vi "DelayProject_WedgeDelay.vi"() -> ()   [LabVIEW 2019]
uses:
  Delete/Control 7.ctl
  Delete/Control 2.ctl
  Delete/Control 1.ctl
  Delete/Control 3.ctl
  Delete/Control 6.ctl
  Delete/Control 4.ctl
  Delete/Control 5.ctl
  Delete/Control 8.ctl
  C:/DATA/Megan/LabviewScripts/ThorlabsKinesisDrivers/Thorlabs.MotionControl.TCube.DCServoCLI.dll
  Thorlabs.MotionControl.TCube.DCServoCLI.dll
  C:/DATA/Megan/LabviewScripts/ThorlabsKinesisDrivers/Thorlabs.MotionControl.Controls.dll
  Thorlabs.MotionControl.Controls.dll
  Program Files (x86)/National Instruments/LabVIEW 2011/user.lib/Nanonis Prog Interface/Nanonis Prog Interface.lvlib
panel:
  in  "TCubeDCServoControl":refnum<k24>(container)
  in  "Start Move B":bool
  in  "Set Position B (mm)":T1 format="%.3f"
  in  "Clear Plots":bool
  in  "Data3":dbl[][](array[numeric])
  out "AFM":cluster{dbl[], dbl[]}[](graph)
  in  "Data2":dbl[][](array[numeric])
  in  "Data1":dbl[][](array[numeric])
  in  "Plot3":bool
  in  "Plot2":bool
  in  "Plot1":bool
  out "Optics":cluster{dbl[], dbl[]}[](graph)
  out "Array":string[][](array[string])
  in  "AC bias (Hz)":string
  in  "AC bias":string
  in  "DC bias":string
  in  "Tip lift":string
  in  "Time const":string
  in  "Prop gain":string
  in  "Polarization":string
  in  "Notes":string
  in  "Location":string
  out "AC bias (Hz)":string="AC Bias (Hz)"
  out "AC bias":string="AC Bias (V)"
  out "DC bias":string="DC Bias (V)"
  out "Polarization":string="Polarization (deg)"
  out "Tip Lift":string="Tip Lift"
  out "Notes":string="Notes"
  out "Location":string="Location"
  out "Time Const":string="Time constant (s)"
  out "Prop Gain":string="Proportional gain (m/Hz)"
  in  "Net Power":string
  in  "Wavelength":string
  out "Net Power":string="Net power (mW)"
  out "Wavelength":string="Wavelength (nm)"
  out "Instantaneous":dbl
  in  "Channel":dbl
  out "Average":dbl
  in  "Wait After (ms)":T2=100.0
  in  "Wait Before (ms)":T3=100.0
  in  "Points per Step":T4=10.0
  in  "Save Sweep":bool
  out "Total Time (min:sec)":string
  out "Range (fs)":dbl
  out "Total Distance (mm)":dbl
  in  "Step Size (mm)":T5 format="%.4f"
  in  "Start Position (mm)":T6=80.0
  in  "End Position (mm)":T7=90.0
  out "Step Size (fs)":dbl=100.0
  out "Status":string
  in  "Set Position A (mm)":T8 format="%.3f"
  in  "Start Move A":bool
  in  "Start Sweep":bool
  out "Time Remaining (min:sec)":string
  in  "Stop Sweep":bool
  out "Position  (mm)":ext format="%.3f"
  # "Wedge Delay"
  # "Sweep"
  # "This program moves the MTS50-Z8 translational delay stage either in a single step (Move), or a  stepped sweep (Sweep). \n\nThe sequence of events in the Sweep is as follows:\n1) Home the stage.\n2) Go to the Start Position; wait 1s.\n3) Move by Step Size.\n4)  Wait Before time. \n5) Write Position to Nanonis Output 8.\n6) Read all Nanonis Channels, Points per Step times.\n7) Take the average of these instantaneous readouts.\n8) Wait After time.\n9) Repeat 3-8 for each step. \n10) Save all Nanonis channels and record Attributes in header.\n\nThe Readouts are for this VI display only, to visualize what the program is doing. Channel is the Nanonis channel displayed. \n\nIf the Set/Start/End positions are outside of the operating range [-1:50]mm, the Move/Sweep will not execute. Short wait times may lead to errors if  they don't allow time  to move. \n\nThis VI needs to be opened from the project directory. This project and VI need to be in the same directory as the Thorlabs Kinesis folder, and require a 64-bit version of Labview. This program cannot run simultaneously with AirDelay.vi"
  # "Attributes"
  # "Parameters"
  # "Readouts"
  # "Move A"
  # "Move B"
  # "Air Delay: 93.15 mm"
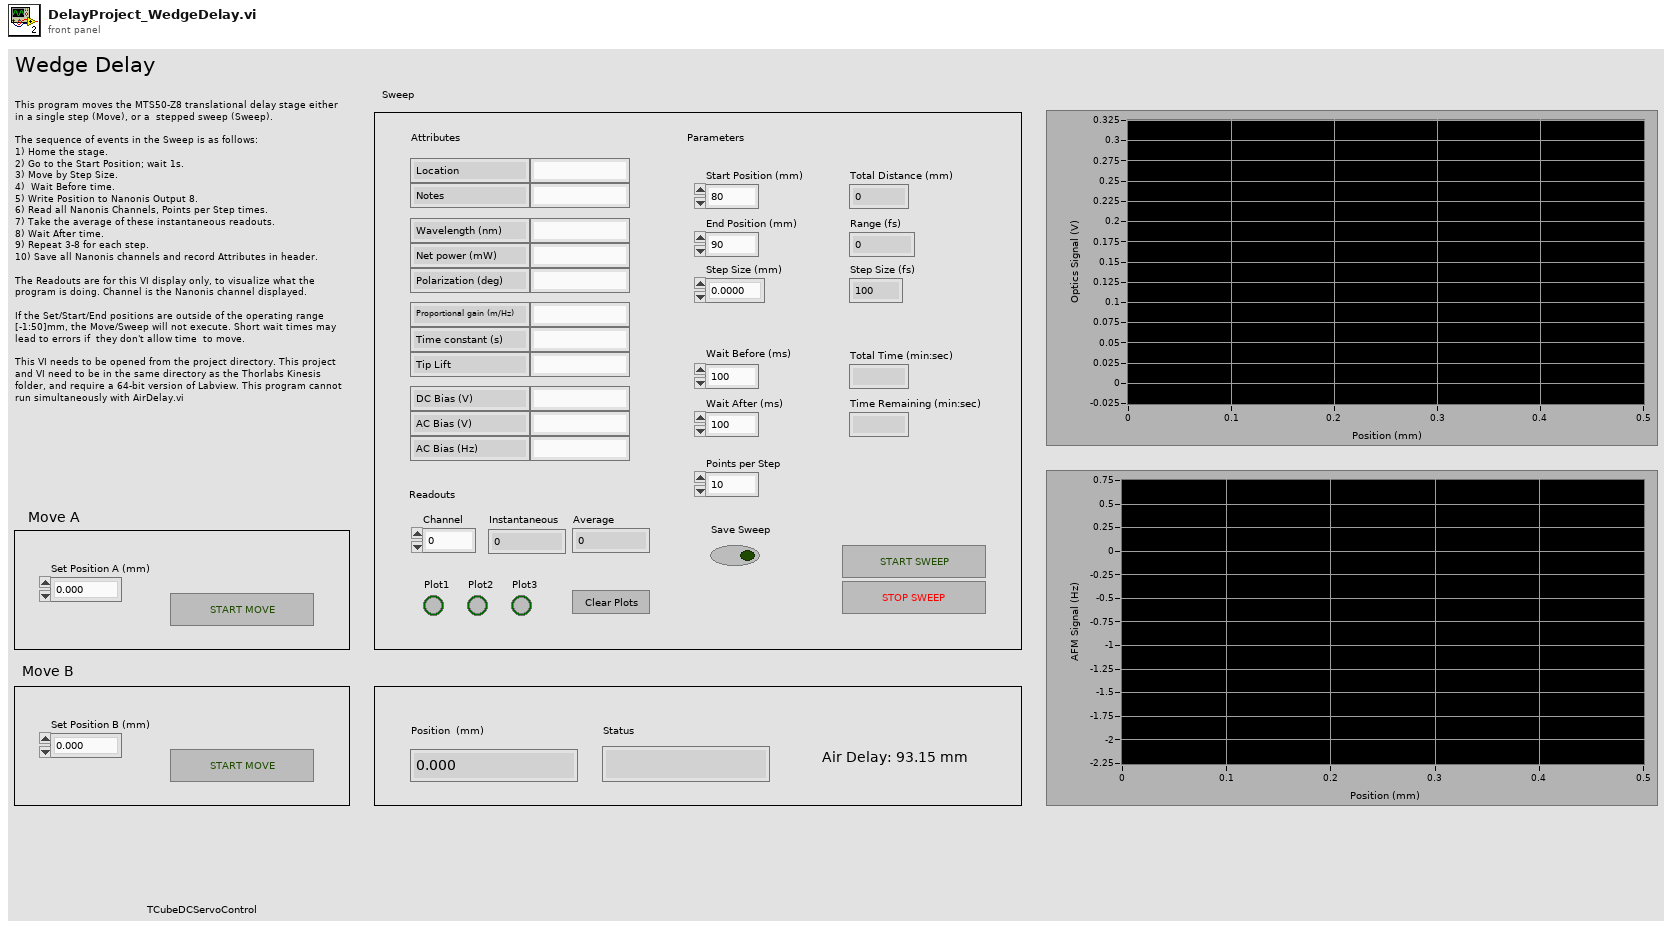
[diagram p1: front panel]
types:
  T1 = typedef "Control 8.ctl" = ext
  T2 = typedef "Control 5.ctl" = dbl
  T3 = typedef "Control 4.ctl" = dbl
  T4 = typedef "Control 6.ctl" = dbl
  T5 = typedef "Control 3.ctl" = dbl
  T6 = typedef "Control 1.ctl" = dbl
  T7 = typedef "Control 2.ctl" = dbl
  T8 = typedef "Control 7.ctl" = ext
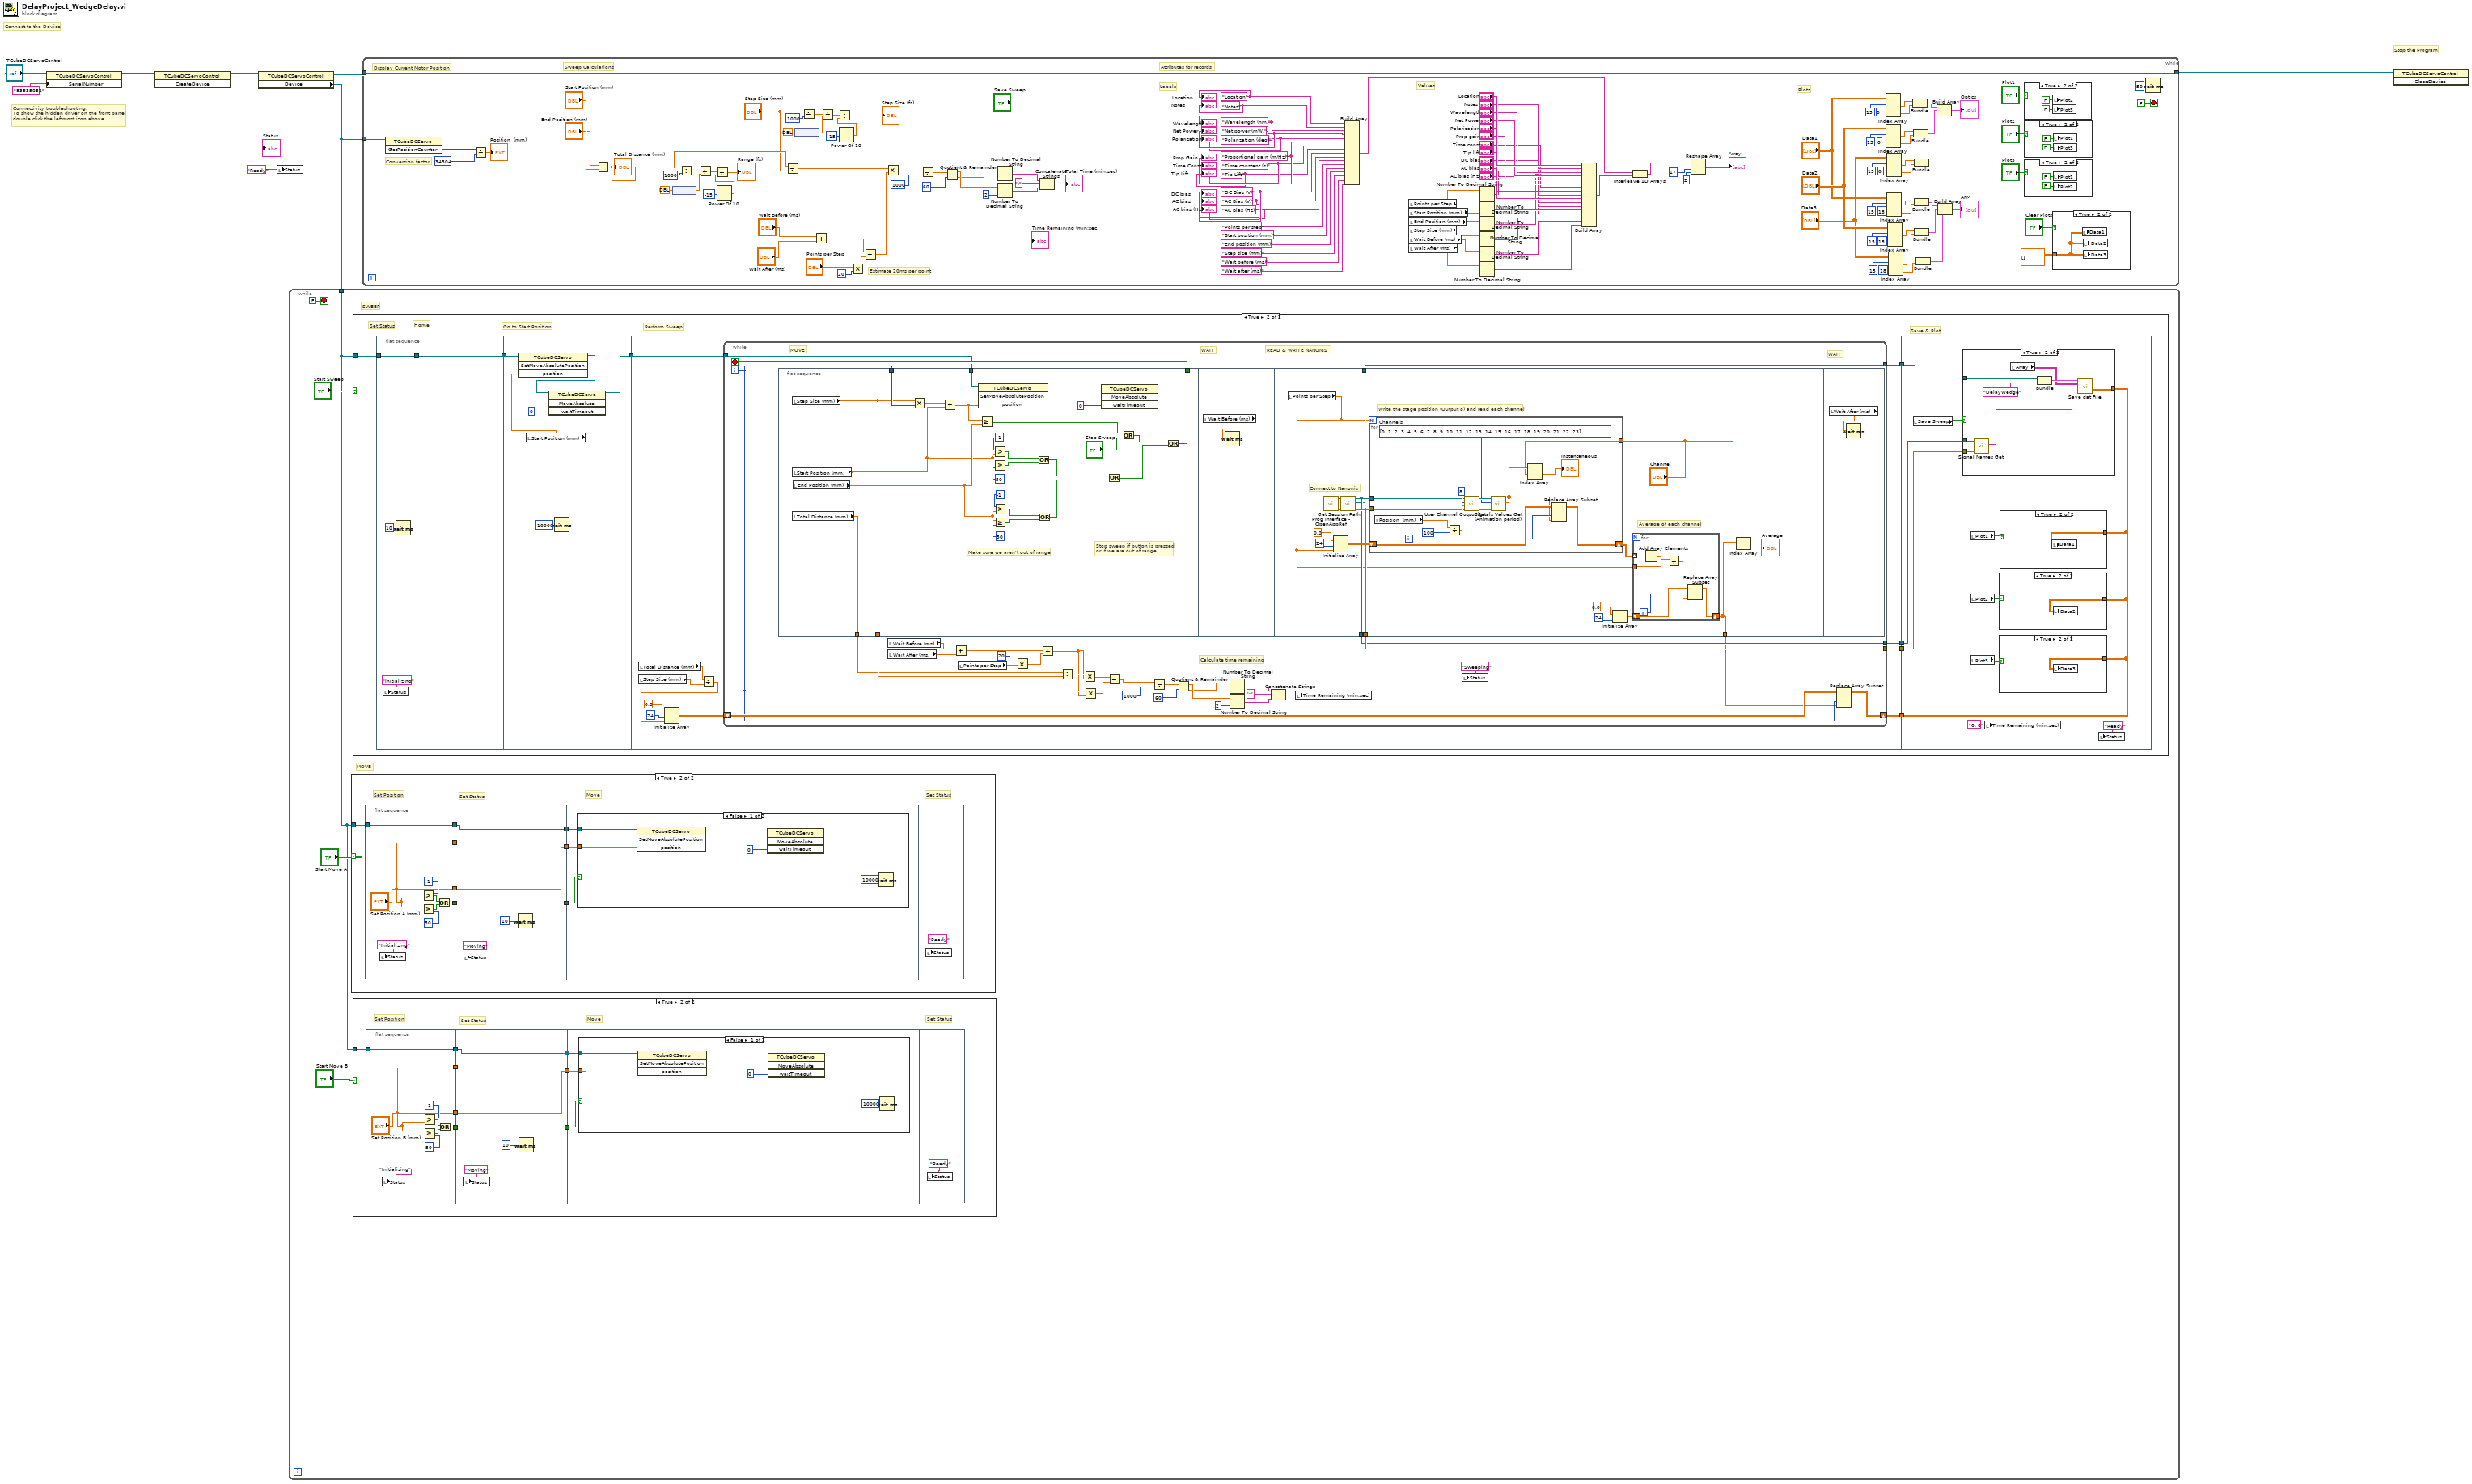
[diagram p0: block diagram]
diagram:
  # "Connectivity troubleshooting: \nTo show the hidden driver on the front panel \ndouble click the leftmost icon above."
  # "Stop the Program"
  # "Connect to the Device"
  n1 = property class="TCubeDCServoControl"(reference="TCubeDCServoControl", "SerialNumber"="83835052") -> (reference out=w8:refnum<k24>)  [unwired: 1 in, 1 out]
  n2 = invoke class="TCubeDCServoControl" method="CreateDevice"(reference=w8) -> (reference out=w5:refnum<k24>)  [unwired: 2 in, 2 out]
  n3 = property class="TCubeDCServoControl"(reference=w5) -> (reference out=w4:refnum<k24>, "Device"=w3:refnum<k24>)  [unwired: 1 in, 1 out]
  n4 = local write "Status"("Ready") -> ()
  n5 = while {
    tunnel: w3 -> [w9]
    stop <- FALSE stop-if-true
    # "MOVE"
    # "SWEEP"
    n6 = case shown="True" "Start Move A" {
      tunnel: w9 -> [_ w51]
      frame False {
      }
      frame True {
        # "Set Status"
        # "Move"
        # "Set Status"
        # "Set Position"
        n7 = flat-sequence {
          tunnel: w51 -> [w59]
          tunnel: [w59] -> w50
          tunnel: ["Set Position A (mm)"] -> w49
          tunnel: [w53] -> w48
          tunnel: ["Set Position A (mm)"] -> w45
          tunnel: w50 -> [w62]
          tunnel: w49 -> [_]
          tunnel: w48 -> [w64]
          tunnel: [w64] -> w47
          tunnel: [w63] -> w46
          tunnel: w45 -> [w63]
          tunnel: [w62] -> w44
          tunnel: w47 -> [w67]
          tunnel: w46 -> [w66]
          tunnel: w44 -> [w65]
          frame #0 {
            n8 = local write "Status"("Initializing") -> ()
            n9 = Greater?(x=-1, y="Set Position A (mm)") -> (0:w58:bool)
            n10 = Greater Or Equal?(x="Set Position A (mm)", y=50) -> (x >= y?=w57:bool)
            n11 = Or(x=w58, y=w57) -> (x .or. y?=w53:bool)
          }
          frame #1 {
            n12 = local write "Status"("Moving") -> ()
            n13 = Wait (ms)(milliseconds to wait=10) -> ()  [unwired: 1 out]
          }
          frame #2 {
            n14 = case shown="False" w67 {
              tunnel: w66 -> [w69 _]
              tunnel: w65 -> [w70 _]
              frame False {
                n15 = invoke class="TCubeDCServo" method="SetMoveAbsolutePosition"(reference=w70, "position"=w69) -> (reference out=w72:refnum<k24>)  [unwired: 2 in, 3 out]
                n16 = invoke class="TCubeDCServo" method="MoveAbsolute"(reference=w72, "waitTimeout"=0) -> ()  [unwired: 2 in, 4 out]
                n17 = Wait (ms)(milliseconds to wait=10000) -> ()  [unwired: 1 out]
              }
              frame True {
              }
            }
          }
          frame #3 {
            n18 = local write "Status"("Ready") -> ()
          }
        }
      }
    }
    n19 = case shown="True" "Start Move B" {
      tunnel: w9 -> [_ w21]
      frame False {
      }
      frame True {
        # "Set Status"
        # "Move"
        # "Set Status"
        # "Set Position"
        n20 = flat-sequence {
          tunnel: w21 -> [w29]
          tunnel: [w29] -> w20
          tunnel: ["Set Position B (mm)"] -> w19
          tunnel: [w24] -> w18
          tunnel: ["Set Position B (mm)"] -> w15
          tunnel: w20 -> [w32]
          tunnel: w19 -> [_]
          tunnel: w18 -> [w34]
          tunnel: [w34] -> w17
          tunnel: [w33] -> w16
          tunnel: w15 -> [w33]
          tunnel: [w32] -> w14
          tunnel: w17 -> [w37]
          tunnel: w16 -> [w36]
          tunnel: w14 -> [w35]
          frame #0 {
            n21 = local write "Status"("Initializing") -> ()
            n22 = Greater?(x=-1, y="Set Position B (mm)") -> (0:w28:bool)
            n23 = Greater Or Equal?(x="Set Position B (mm)", y=50) -> (x >= y?=w27:bool)
            n24 = Or(x=w28, y=w27) -> (x .or. y?=w24:bool)
          }
          frame #1 {
            n25 = local write "Status"("Moving") -> ()
            n26 = Wait (ms)(milliseconds to wait=10) -> ()  [unwired: 1 out]
          }
          frame #2 {
            n27 = case shown="False" w37 {
              tunnel: w36 -> [w39 _]
              tunnel: w35 -> [w40 _]
              frame False {
                n28 = invoke class="TCubeDCServo" method="SetMoveAbsolutePosition"(reference=w40, "position"=w39) -> (reference out=w42:refnum<k24>)  [unwired: 2 in, 3 out]
                n29 = invoke class="TCubeDCServo" method="MoveAbsolute"(reference=w42, "waitTimeout"=0) -> ()  [unwired: 2 in, 4 out]
                n30 = Wait (ms)(milliseconds to wait=10000) -> ()  [unwired: 1 out]
              }
              frame True {
              }
            }
          }
          frame #3 {
            n31 = local write "Status"("Ready") -> ()
          }
        }
      }
    }
    n32 = case shown="True" "Start Sweep" {
      tunnel: w9 -> [_ w81]
      frame False {
      }
      frame True {
        # "Save & Plot"
        # "Set Status"
        # "Perform Sweep"
        # "Go to Start Position"
        # "Home"
        n33 = flat-sequence {
          tunnel: w81 -> [w84]
          tunnel: [w84] -> w80
          tunnel: [w85] -> w79
          tunnel: w80 -> [w85]
          tunnel: w79 -> [w91]
          tunnel: [w88] -> w78
          tunnel: w78 -> [w102]
          tunnel: [w101] -> w77
          tunnel: [w100] -> w76
          tunnel: [w99] -> w75
          tunnel: [w92] -> w74
          tunnel: w77 -> [w208]
          tunnel: w76 -> [w207]
          tunnel: w75 -> [w206]
          tunnel: w74 -> [w204]
          frame #0 {
            n34 = local write "Status"("Initializing") -> ()
            n35 = Wait (ms)(milliseconds to wait=10) -> ()  [unwired: 1 out]
          }
          frame #1 {
          }
          frame #2 {
            n36 = local read "Start Position (mm)"() -> (w86:T6)
            n37 = invoke class="TCubeDCServo" method="SetMoveAbsolutePosition"(reference=w91, "position"=w86) -> (reference out=w89:refnum<k24>)  [unwired: 2 in, 3 out]
            n38 = invoke class="TCubeDCServo" method="MoveAbsolute"(reference=w89, "waitTimeout"=0) -> (reference out=w88:refnum<k24>)  [unwired: 2 in, 3 out]
            n39 = Wait (ms)(milliseconds to wait=10000) -> ()  [unwired: 1 out]
          }
          frame #3 {
            n40 = local read "Total Distance (mm)"() -> (w96:dbl)
            n41 = local read "Step Size (mm)"() -> (w95:T5)
            n42 = Divide(x=w96, y=w95) -> (x/y=w94:T5)
            n43 = Initialize Array(0.0, 24, w94) -> (w93:dbl[][])
            n44 = while {
              tunnel: w102 -> [w134]
              tunnel: [w114] -> w101
              tunnel: [w115] -> w100
              tunnel: [w113] -> w99
              shift-right: [w109] -> w92
              shift-left: w93 -> [w112]
              i -> [w111]
              stop <- w135 stop-if-true
              # "WAIT"
              # "READ & WRITE NANONIS"
              # "WAIT"
              # "MOVE"
              # "Calculate time remaining"
              n45 = flat-sequence {
                tunnel: w111 -> [w140]
                tunnel: [w139] -> w135
                tunnel: w134 -> [w138]
                tunnel: [w137] -> w124
                tunnel: [w136] -> w123
                tunnel: [w167] -> w115
                tunnel: [w166] -> w114
                tunnel: [w165] -> w113
                tunnel: [w164] -> w110
                frame #0 {
                  # "Stop sweep if button is pressed\nor if we are out of range"
                  # "Make sure we aren't out of range"
                  n46 = local read "Step Size (mm)"() -> (w137:T5)
                  n47 = local read "Start Position (mm)"() -> (w159:T6)
                  n48 = local read "Total Distance (mm)"() -> (w136:dbl)
                  n49 = local read "End Position (mm)"() -> (w160:T7)
                  n50 = Multiply(x=w137, y=w140) -> (x*y=w145:T5)
                  n51 = Add(x=w145, y=w159) -> (x+y=w146:T5)
                  n52 = invoke class="TCubeDCServo" method="SetMoveAbsolutePosition"(reference=w138, "position"=w146) -> (reference out=w141:refnum<k24>)  [unwired: 2 in, 3 out]
                  n53 = Greater Or Equal?(x=w146, y=w160) -> (x >= y?=w144:bool)
                  n54 = Greater?(x=-1, y=w159) -> (0:w151:bool)
                  n55 = Greater Or Equal?(x=w159, y=50) -> (x >= y?=w152:bool)
                  n56 = Greater?(x=-1, y=w160) -> (0:w155:bool)
                  n57 = Greater Or Equal?(x=w160, y=50) -> (x >= y?=w156:bool)
                  n58 = Or(x=w151, y=w152) -> (x .or. y?=w157:bool)
                  n59 = Or(x=w155, y=w156) -> (x .or. y?=w158:bool)
                  n60 = invoke class="TCubeDCServo" method="MoveAbsolute"(reference=w141, "waitTimeout"=0) -> ()  [unwired: 2 in, 4 out]
                  n61 = Or(x=w157, y=w158) -> (x .or. y?=w148:bool)
                  n62 = Or(x=w144, y="Stop Sweep") -> (x .or. y?=w147:bool)
                  n63 = Or(x=w147, y=w148) -> (x .or. y?=w139:bool)
                }
                frame #1 {
                  n64 = local read "Wait Before (ms)"() -> (w161:T3)
                  n65 = Wait (ms)(milliseconds to wait=w161) -> ()  [unwired: 1 out]
                }
                frame #2 {
                  # "Write the stage position (Output 8) and read each channel"
                  # "Average of each channel"
                  # "Connect to Nanonis"
                  n66 = local read "Points per Step"() -> (w163:T4)
                  n67 = call "Prog Interface - OpenAppRef.vi"() -> ("Error out"=w168:errorcluster, "Application reference"=w169:refnum<vi>)  [unwired: 6 in]
                  n68 = Initialize Array(0.0, 24, w163) -> (w172:dbl[][])
                  n69 = call "Get Session Path.vi"("error in (no error)"=w168, "Application ref in"=w169) -> ("error out"=w167:errorcluster, "Session path"=w165:path, "Application ref out"=w166:refnum<vi>)  [unwired: 7 in]
                  n70 = for {
                    N: w163 -> [_]
                    tunnel: w167 -> [w193]
                    tunnel: w166 -> [w192]
                    shift-right: [w191] -> w176
                    shift-left: w172 -> [w190]
                    tunnel: "Channel" -> [w185]
                    i -> [w189]
                    w186 = i32[] [0, 1, 2, 3, 4, 5, 6, 7, 8, 9, 10, 11, 12, 13, 14, 15, 16, 17, 18, 19, 20, 21, 22, 23]  # Channels
                    n71 = local read "Position  (mm)"() -> (w187:ext)
                    n72 = Divide(x=w187, y=100) -> (x/y=w196:ext)
                    n73 = call "User Channel Output Set.vi"("error in (no error)"=w193, "Output value (physical unit)"=w196, "User output channel (1-8)"=8, "Application ref in"=w192) -> ("error out"=w198:errorcluster, "Application ref out"=w197:refnum<vi>)  [unwired: 5 in]
                    n74 = call "Signals Values Get (Animation period).vi"("error in (no error)"=w198, "Signals indexes (0-23)"=w186, "Application ref in"=w197) -> ("Signals Values"=w188:sgl[])  [unwired: 5 in, 2 out]
                    n75 = Index Array(array=w188, index #1=w185) -> (element #1=→"Instantaneous":sgl)  [unwired: 1 in, 1 out]
                    n76 = Replace Array Subset(array=w190, new element=w188, index (col)=w189) -> (w191:dbl[][])  [unwired: 1 in]
                  }
                  n77 = Initialize Array(0.0, 24) -> (w175:dbl[])
                  n78 = for {
                    tunnel: w163 -> [w184]
                    tunnel: w176 -> [w180] mode=indexing
                    shift-right: [w182] -> w164
                    shift-left: w175 -> [w183]
                    i -> [w181]
                    n79 = Add Array Elements(numeric array=w180) -> (sum=w178:dbl)
                    n80 = Divide(x=w178, y=w184) -> (x/y=w179:T4)
                    n81 = Replace Array Subset(array=w183, new element=w179, index=w181) -> (w182:dbl[])
                  }
                  n82 = Index Array(array=w164, index="Channel") -> (element=→"Average":dbl)
                }
                frame #3 {
                  n83 = local read "Wait After (ms)"() -> (w200:T2)
                  n84 = Wait (ms)(milliseconds to wait=w200) -> ()  [unwired: 1 out]
                }
              }
              n85 = local read "Wait Before (ms)"() -> (w117:T3)
              n86 = local read "Wait After (ms)"() -> (w116:T2)
              n87 = Add(x=w117, y=w116) -> (x+y=w107:T3)
              n88 = local read "Points per Step"() -> (w108:T4)
              n89 = Multiply(x=20, y=w108) -> (x*y=w105:T4)
              n90 = Add(x=w107, y=w105) -> (x+y=w106:T3)
              n91 = Divide(x=w123, y=w124) -> (x/y=w125:T5)
              n92 = Multiply(x=w125, y=w106) -> (x*y=w126:T5)
              n93 = Multiply(x=w111, y=w106) -> (x*y=w128:T3)
              n94 = Subtract(x=w126, y=w128) -> (x-y=w127:T5)
              n95 = Divide(x=w127, y=1000) -> (x/y=w133:T5)
              n96 = Quotient & Remainder(x=w133, y=60) -> (x-y*floor(x/y)=w132:T5, floor(x/y)=w131:T5)
              n97 = Number To Decimal String(number=w131) -> (decimal integer string=w130:string)  [unwired: 1 in]
              n98 = Number To Decimal String(number=w132, width (-)=2) -> (decimal integer string=w129:string)
              n99 = Concatenate Strings(w130, ":", w129) -> (w103:string)
              n100 = local write "Time Remaining (min:sec)"(w103) -> ()
              n101 = local write "Status"("Sweeping") -> ()
              n102 = Replace Array Subset(array=w112, new element=w110, index (col)=w111) -> (w109:dbl[][])  [unwired: 1 in]
            }
          }
          frame #4 {
            n103 = local read "Save Sweep"() -> (w209:bool)
            n104 = case shown="True" w209 {
              tunnel: w207 -> [_ w219]
              tunnel: w208 -> [_ w218]
              tunnel: w206 -> [_ w216]
              tunnel: w204 -> [_ w215]
              frame False {
              }
              frame True {
                n105 = call "Signal Names Get.vi"("error in (no error)"=w219, "Application ref in"=w218) -> ("Signals Names"=w217:string[])  [unwired: 5 in, 2 out]
                n106 = local read "Array"() -> (w214:string[][])
                n107 = Bundle("Session path"=w216, "DelayWedge") -> (w221:cluster{"Session path":path, string})  [unwired: 1 in]
                n108 = call "Save dat File.vi"("Filename control"=w221, "Attributes"=w214, "Channels names"=w217, "Data"=w215) -> ()  [unwired: 8 in, 4 out]
              }
            }
            n109 = local read "Plot1"() -> (w201:bool)
            n110 = local read "Plot2"() -> (w202:bool)
            n111 = local read "Plot3"() -> (w203:bool)
            n112 = local write "Time Remaining (min:sec)"("0: 0") -> ()
            n113 = case shown="True" w202 {
              tunnel: w204 -> [_ w212]
              frame False {
              }
              frame True {
                n114 = local write "Data2"(w212) -> ()
              }
            }
            n115 = case shown="True" w203 {
              tunnel: w204 -> [_ w211]
              frame False {
              }
              frame True {
                n116 = local write "Data3"(w211) -> ()
              }
            }
            n117 = case shown="True" w201 {
              tunnel: w204 -> [_ w213]
              frame False {
              }
              frame True {
                n118 = local write "Data1"(w213) -> ()
              }
            }
            n119 = local write "Status"("Ready") -> ()
          }
        }
      }
    }
  }
  n120 = while {
    tunnel: [w353] -> w7
    tunnel: w4 -> [w353]
    tunnel: w3 -> [w222]
    stop <- FALSE stop-if-true
    w276 = "Polarization (deg)"
    w279 = "Notes"
    w280 = "Location"
    w273 = "Tip Lift"
    w270 = "AC Bias (Hz)"
    w271 = "AC Bias (V)"
    w272 = "DC Bias (V)"
    w274 = "Time constant (s)"
    w275 = "Proportional gain (m/Hz)"
    w277 = "Net power (mW)"
    w278 = "Wavelength (nm)"
    # "Plots"
    # "Estimate 20ms per point"
    # "Values"
    # "Labels"
    # "Attributes for records"
    # "Sweep Calculations"
    # "Display Current Motor Position"
    # "Conversion factor"
    n121 = invoke class="TCubeDCServo" method="GetPositionCounter"(reference=w222) -> ("GetPositionCounter"=w352:i32)  [unwired: 2 in, 2 out]
    n122 = Divide(x=w352, y=34304) -> (x/y=→"Position  (mm)":dbl)
    n123 = Subtract(x="End Position (mm)", y="Start Position (mm)") -> (x-y=w320:T7)
    "Total Distance (mm)" <- w320
    n124 = node(ext[unit] 299792458.0) -> (w336:ext)
    n125 = Divide(x=w320, y=1000) -> (x/y=w337:T7)
    n126 = Divide(x=w337, y=w336) -> (x/y=w335:ext)
    n127 = Power Of 10(x=-15) -> (10^x=w332:dbl)
    n128 = Divide(x=w335, y=w332) -> (x/y=→"Range (fs)":ext)
    n129 = Divide(x=w320, y="Step Size (mm)") -> (x/y=w317:T7)
    n130 = node(ext[unit] 299792458.0) -> (w346:ext)
    n131 = Divide(x="Step Size (mm)", y=1000) -> (x/y=w345:T5)
    n132 = Add(x="Wait Before (ms)", y="Wait After (ms)") -> (x+y=w268:T3)
    n133 = Divide(x=w345, y=w346) -> (x/y=w347:ext)
    n134 = Power Of 10(x=-15) -> (10^x=w348:dbl)
    n135 = Divide(x=w347, y=w348) -> (x/y=→"Step Size (fs)":ext)
    n136 = Multiply(x="Points per Step", y=20) -> (x*y=w269:T4)
    n137 = Add(x=w268, y=w269) -> (x+y=w267:T3)
    n138 = Multiply(x=w317, y=w267) -> (x*y=w321:T7)
    n139 = Divide(x=w321, y=1000) -> (x/y=w329:T7)
    n140 = Quotient & Remainder(x=w329, y=60) -> (x-y*floor(x/y)=w327:T7, floor(x/y)=w326:T7)
    n141 = Number To Decimal String(number=w326) -> (decimal integer string=w325:string)  [unwired: 1 in]
    n142 = Number To Decimal String(number=w327, width (-)=2) -> (decimal integer string=w323:string)
    n143 = Concatenate Strings(w325, ":", w323) -> (→"Total Time (min:sec)":string)
    n144 = Build Array(w280, w279, w278, w277, w276, w275, w274, w273, w272, w271, w270, "Points per step", "Start position (mm)", "End position (mm)", "Step size (mm)", "Wait before (ms)", "Wait after (ms)") -> (w284:string[])
    n145 = local read "Points per Step"() -> (w314:T4)
    n146 = local read "Start Position (mm)"() -> (w313:T6)
    n147 = local read "End Position (mm)"() -> (w312:T7)
    n148 = local read "Step Size (mm)"() -> (w311:T5)
    n149 = local read "Wait Before (ms)"() -> (w310:T3)
    n150 = local read "Wait After (ms)"() -> (w309:T2)
    n151 = Number To Decimal String(number=w314) -> (decimal integer string=w296:string)  [unwired: 1 in]
    n152 = Number To Decimal String(number=w313) -> (decimal integer string=w295:string)  [unwired: 1 in]
    n153 = Number To Decimal String(number=w312) -> (decimal integer string=w294:string)  [unwired: 1 in]
    n154 = Number To Decimal String(number=w311) -> (decimal integer string=w293:string)  [unwired: 1 in]
    n155 = Number To Decimal String(number=w310) -> (decimal integer string=w292:string)  [unwired: 1 in]
    n156 = Number To Decimal String(number=w309) -> (decimal integer string=w285:string)  [unwired: 1 in]
    n157 = Build Array("Location", "Notes", "Wavelength", "Net Power", "Polarization", "Prop gain", "Time const", "Tip lift", "DC bias", "AC bias", "AC bias (Hz)", w296, w295, w294, w293, w292, w285) -> (w283:string[])
    n158 = Interleave 1D Arrays(w284, w283) -> (w282:string[])
    n159 = Reshape Array(w282, 17, 2) -> (→"Array":string[][])
    n160 = Index Array(array="Data1", index (row) #1=15, index (row) #2=0) -> (element #1=w261:dbl[], element #2=w262:dbl[])  [unwired: 2 in]
    n161 = Index Array(array="Data2", index (row) #1=15, index (row) #2=0) -> (element #1=w256:dbl[], element #2=w257:dbl[])  [unwired: 2 in]
    n162 = Index Array(array="Data3", index (row) #1=15, index (row) #2=0) -> (element #1=w252:dbl[], element #2=w253:dbl[])  [unwired: 2 in]
    n163 = Index Array(array="Data1", index (row) #1=15, index (row) #2=18) -> (element #1=w245:dbl[], element #2=w246:dbl[])  [unwired: 2 in]
    n164 = Index Array(array="Data2", index (row) #1=15, index (row) #2=18) -> (element #1=w241:dbl[], element #2=w242:dbl[])  [unwired: 2 in]
    n165 = Index Array(array="Data3", index (row) #1=15, index (row) #2=18) -> (element #1=w237:dbl[], element #2=w238:dbl[])  [unwired: 2 in]
    n166 = Bundle("Data1"=w261, "Data1"=w262) -> (w249:cluster{"Data1":dbl[], "Data1":dbl[]})  [unwired: 1 in]
    n167 = Bundle("Data2"=w256, "Data2"=w257) -> (w248:cluster{"Data2":dbl[], "Data2":dbl[]})  [unwired: 1 in]
    n168 = Bundle("Data3"=w252, "Data3"=w253) -> (w247:cluster{"Data3":dbl[], "Data3":dbl[]})  [unwired: 1 in]
    n169 = Bundle("Data1"=w245, "Data1"=w246) -> (w234:cluster{"Data1":dbl[], "Data1":dbl[]})  [unwired: 1 in]
    n170 = Bundle("Data2"=w241, "Data2"=w242) -> (w233:cluster{"Data2":dbl[], "Data2":dbl[]})  [unwired: 1 in]
    n171 = Bundle("Data3"=w237, "Data3"=w238) -> (w232:cluster{"Data3":dbl[], "Data3":dbl[]})  [unwired: 1 in]
    n172 = Build Array(w249, w248, w247) -> (→"Optics":cluster{"Data3":dbl[], "Data3":dbl[]}[])
    n173 = Build Array(w234, w233, w232) -> (→"AFM":cluster{"Data3":dbl[], "Data3":dbl[]}[])
    n174 = case shown="True" "Plot1" {
      frame False {
      }
      frame True {
        n175 = local write "Plot2"(FALSE) -> ()
        n176 = local write "Plot3"(FALSE) -> ()
      }
    }
    n177 = case shown="True" "Plot2" {
      frame False {
      }
      frame True {
        n178 = local write "Plot1"(FALSE) -> ()
        n179 = local write "Plot3"(FALSE) -> ()
      }
    }
    n180 = case shown="True" "Plot3" {
      frame False {
      }
      frame True {
        n181 = local write "Plot1"(FALSE) -> ()
        n182 = local write "Plot2"(FALSE) -> ()
      }
    }
    n183 = case shown="True" "Clear Plots" {
      tunnel: dbl[][] [] ("Plot 3") -> [_ w360]
      frame False {
      }
      frame True {
        n184 = local write "Data1"(w360) -> ()
        n185 = local write "Data2"(w360) -> ()
        n186 = local write "Data3"(w360) -> ()
      }
    }
    n187 = Wait (ms)(milliseconds to wait=50) -> ()  [unwired: 1 out]
    "Wavelength" <- w278
    "Net Power" <- w277
    "Prop Gain" <- w275
    "Time Const" <- w274
    "Location" <- w280
    "Notes" <- w279
    "Tip Lift" <- w273
    "Polarization" <- w276
    "DC bias" <- w272
    "AC bias" <- w271
    "AC bias (Hz)" <- w270
  }
  n188 = invoke class="TCubeDCServoControl" method="CloseDevice"(reference=w7) -> ()  [unwired: 2 in, 3 out]
